vi "Caliper Setting UI.vi"(7 "Coor?":bool, 8 "error in (no error)":errorcluster, 9 "CaliperEntryIn Overlay In":T2[](array[typedef]) {"CaliperType" items=["Distance", "Mid Point", "Perpendicular Projection", "Lines Intersection", "Angle from Horizontal", "Angle from Vertical", "Angle Defined by 3 Points", "Angle Defined by 4 Points", "Bissecting Line", "Mid Line", "Center of Mass", "Area", "Line Fit", "Circle Fit", "Ellipse Fit"]}, 10 "CaliperEntryIn":T2[](array[typedef]) {"CaliperType" items=["Distance", "Mid Point", "Perpendicular Projection", "Lines Intersection", "Angle from Horizontal", "Angle from Vertical", "Angle Defined by 3 Points", "Angle Defined by 4 Points", "Bissecting Line", "Mid Line", "Center of Mass", "Area", "Line Fit", "Circle Fit", "Ellipse Fit"]}, 11 "Vision_Image":T7(plugin-control)) -> (0 "error out":errorcluster, 1 "CaliperEntryOut Overlay":T2[](array[typedef]) {"CaliperType" items=["Distance", "Mid Point", "Perpendicular Projection", "Lines Intersection", "Angle from Horizontal", "Angle from Vertical", "Angle Defined by 3 Points", "Angle Defined by 4 Points", "Bissecting Line", "Mid Line", "Center of Mass", "Area", "Line Fit", "Circle Fit", "Ellipse Fit"]}, 2 "CaliperEntryOut":T2[](array[typedef]) {"CaliperType" items=["Distance", "Mid Point", "Perpendicular Projection", "Lines Intersection", "Angle from Horizontal", "Angle from Vertical", "Angle Defined by 3 Points", "Angle Defined by 4 Points", "Bissecting Line", "Mid Line", "Center of Mass", "Area", "Line Fit", "Circle Fit", "Ellipse Fit"]}, 3 "Cancel?":bool)   [LabVIEW 2019]
uses:
  Controls/CaliperType with Picture.ctl
  Controls/SelectionListEntry.ctl
  Controls/SelectionListEntryPointType.ctl
  Controls/CaliperDataEntry.ctl
  Controls/CaliperType.ctl
  Controls/CaliperResult.ctl
  Controls/Caliper_UI_Action.ctl
  Controls/AnalysisResultPointsAction.ctl
  Analysis/Controls/Analysis_Result_To_Caliper.ctl
  <vilib>/vision/NI_Vision_Development_Module.lvlib
panel:
  out "Result Overlay":T1
  out "CaliperEntryList Overlay":T2[](array[typedef]) {"CaliperType" items=["Distance", "Mid Point", "Perpendicular Projection", "Lines Intersection", "Angle from Horizontal", "Angle from Vertical", "Angle Defined by 3 Points", "Angle Defined by 4 Points", "Bissecting Line", "Mid Line", "Center of Mass", "Area", "Line Fit", "Circle Fit", "Ellipse Fit"]}
  in  "Run All":bool
  in  "ReplaceCaliper":bool
  out "Result":string
  in  "DeleteCaliper":bool
  in  "CaliperList":i32(listbox)=-1
  in  "AddCaliper":bool
  out "Result":T1
  out "CaliperEntryList":T2[](array[typedef]) {"CaliperType" items=["Distance", "Mid Point", "Perpendicular Projection", "Lines Intersection", "Angle from Horizontal", "Angle from Vertical", "Angle Defined by 3 Points", "Angle Defined by 4 Points", "Bissecting Line", "Mid Line", "Center of Mass", "Area", "Line Fit", "Circle Fit", "Ellipse Fit"]}
  out "AnalysisResultNum":i32
  out "SelectionList":T4[](array[typedef])
  out "Row":i32
  out "Analysis Results":i32[](listbox)
  in  "CaliperType_w_Pic":T6 items=["Distance", "Mid Point", "Perpendicular Projection", "Lines Intersection", "Angle from Horizontal", "Angle from Vertical", "Angle Defined by 3 Points", "Angle Defined by 4 Points", "Bissecting Line", "Mid Line", "Area", "Line Fit", "Circle Fit"]
  in  "Cancel":bool
  in  "Done":bool
  in  "Run Algorithm":bool
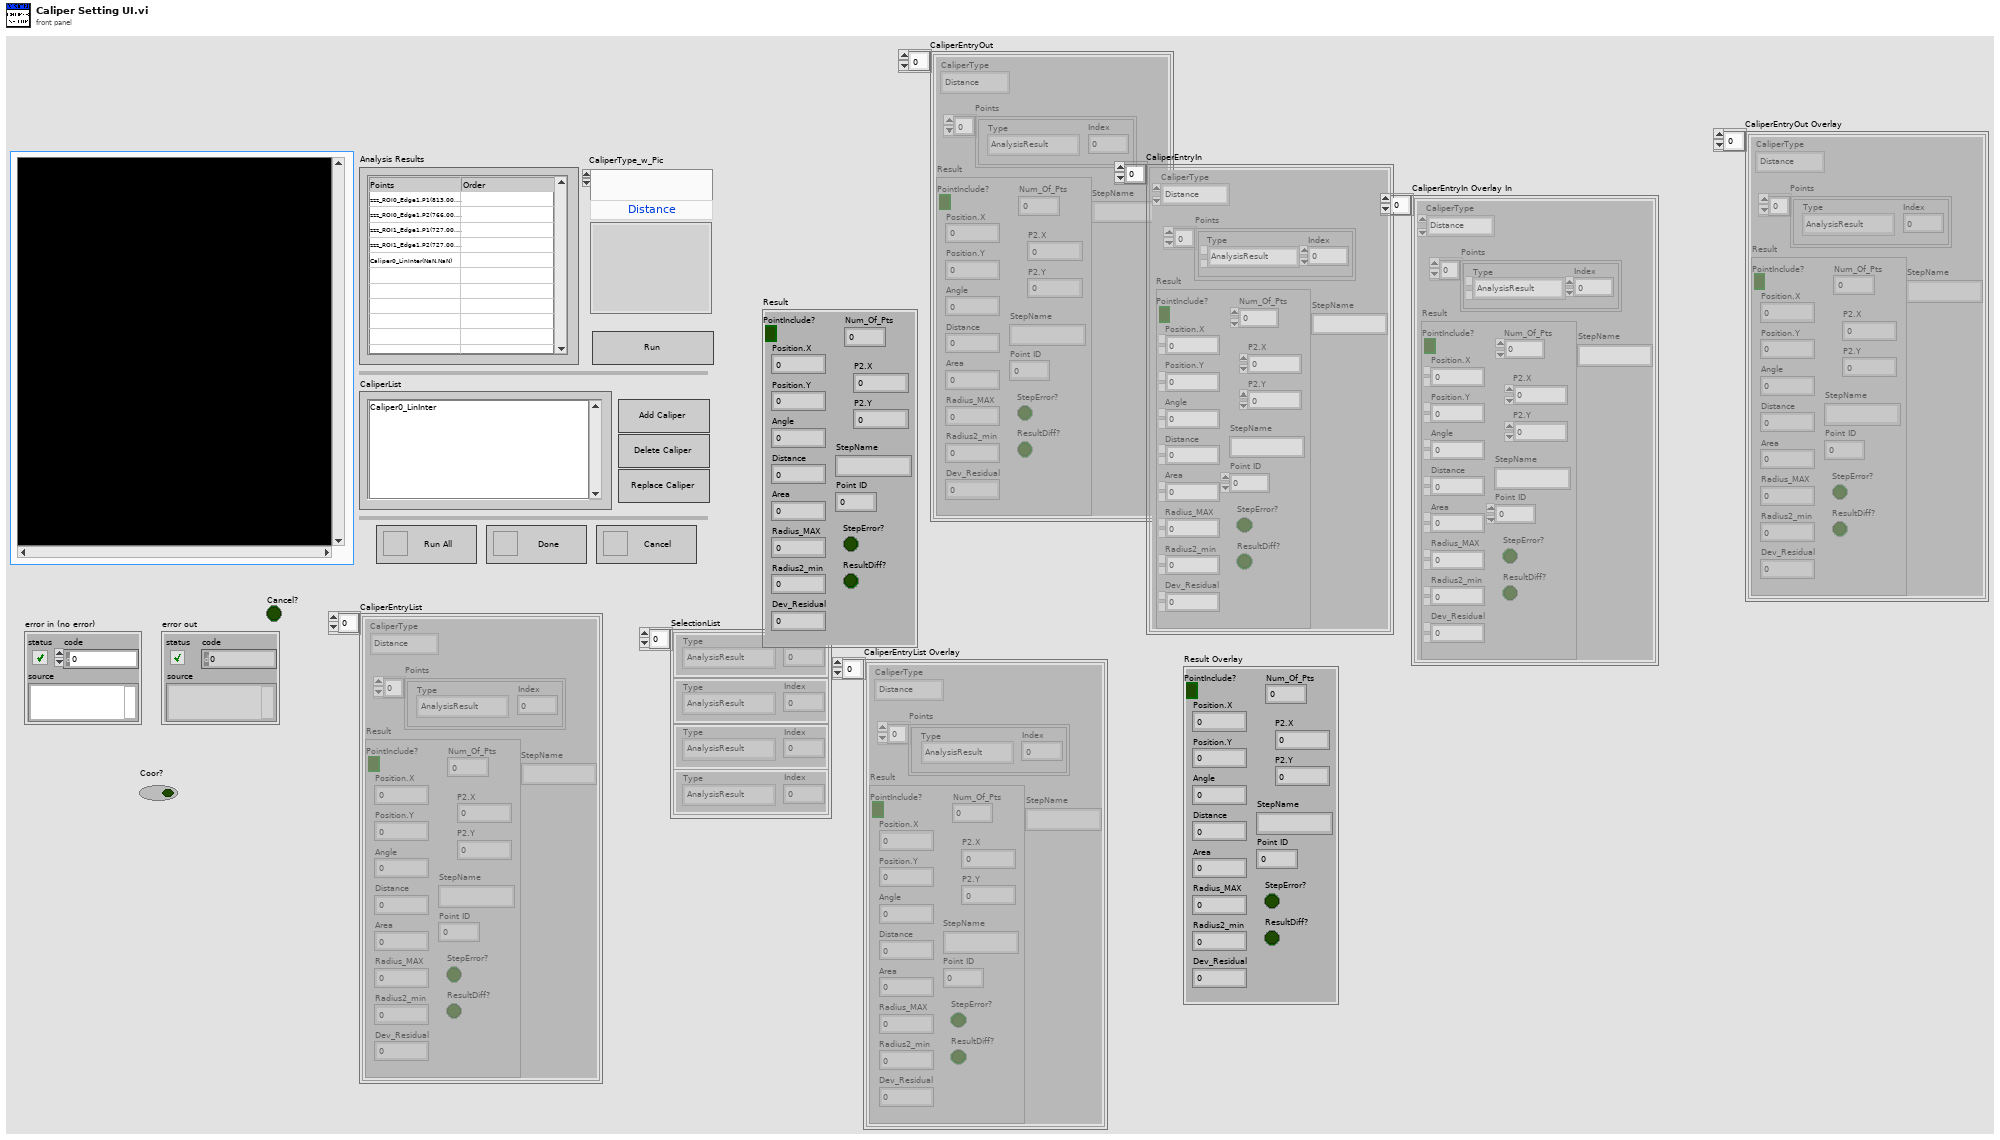
[diagram p1: front panel]
types:
  T1 = typedef "CaliperResult.ctl" = cluster{"PointInclude?":bool, "Num_Of_Pts":u8, "Position.X":dbl, "Position.Y":dbl, "Angle":dbl, "Distance":dbl, "Area":dbl, "Radius_MAX":dbl, "Radius2_min":dbl, "Dev_Residual":dbl, "P2.X":dbl, "P2.Y":dbl, "StepName":string, "Point ID":u8, "StepError?":bool, "ResultDiff?":bool}
  T2 = typedef "CaliperDataEntry.ctl" = cluster{"CaliperType":T3, "Points":T4[], "Result":T1, "StepName":string}
  T3 = typedef "CaliperType.ctl" = u32
  T4 = typedef "SelectionListEntry.ctl" = cluster{"Type":T5, "Index":i32}
  T5 = typedef "SelectionListEntryPointType.ctl" = enum16{"AnalysisResult", "CaliperResult"}
  T6 = typedef "CaliperType with Picture.ctl" = u32
  T7 = typedef "IMAQ Image.ctl" = refnum<image>
  T8 = typedef "Caliper_UI_Action.ctl" = enum16{"Init", "Done", "Cancel", "Run", "InitAnalysisResultTable", "UpdateSymbol", "UpdateOrderInTable", "UpdateAnalysisTable", "UpdateCaliperResultToTable", "AddCaliperEntry", "SetCaliperStepName", "UpdateCaliperList", "RemoveCaliperEntry", "ResetSelectionList", "ReplaceCaliperEntry", "RunAll", "Updata Overlay", "Clean Overlay"}
  T9 = typedef "Analysis_Result_To_Caliper.ctl" = cluster{"PointName":string, "Position_X":dbl, "Position_Y":dbl}
  T10 = typedef "AnalysisResultPointsAction.ctl" = enum16{"Init", "Add", "Delete", "ReplaceAll", "ReadAll", "Close"}
  T11 = typedef "CaliperDataEntry_SinglePoint.ctl" = cluster{"CaliperType":T3, "Points":T4[], "Result":T12, "StepName":string}
  T12 = typedef "CaliperResult_SinglePoint.ctl" = cluster{"PointInclude?":bool, "Position.X":dbl, "Position.Y":dbl, "Angle":dbl, "Distance":dbl, "Area":dbl, "Radius_MAX":dbl, "Radius2_min":dbl, "Dev_Residual":dbl, "StepName":string, "Point ID":u8, "StepError?":bool, "ResultDiff?":bool}
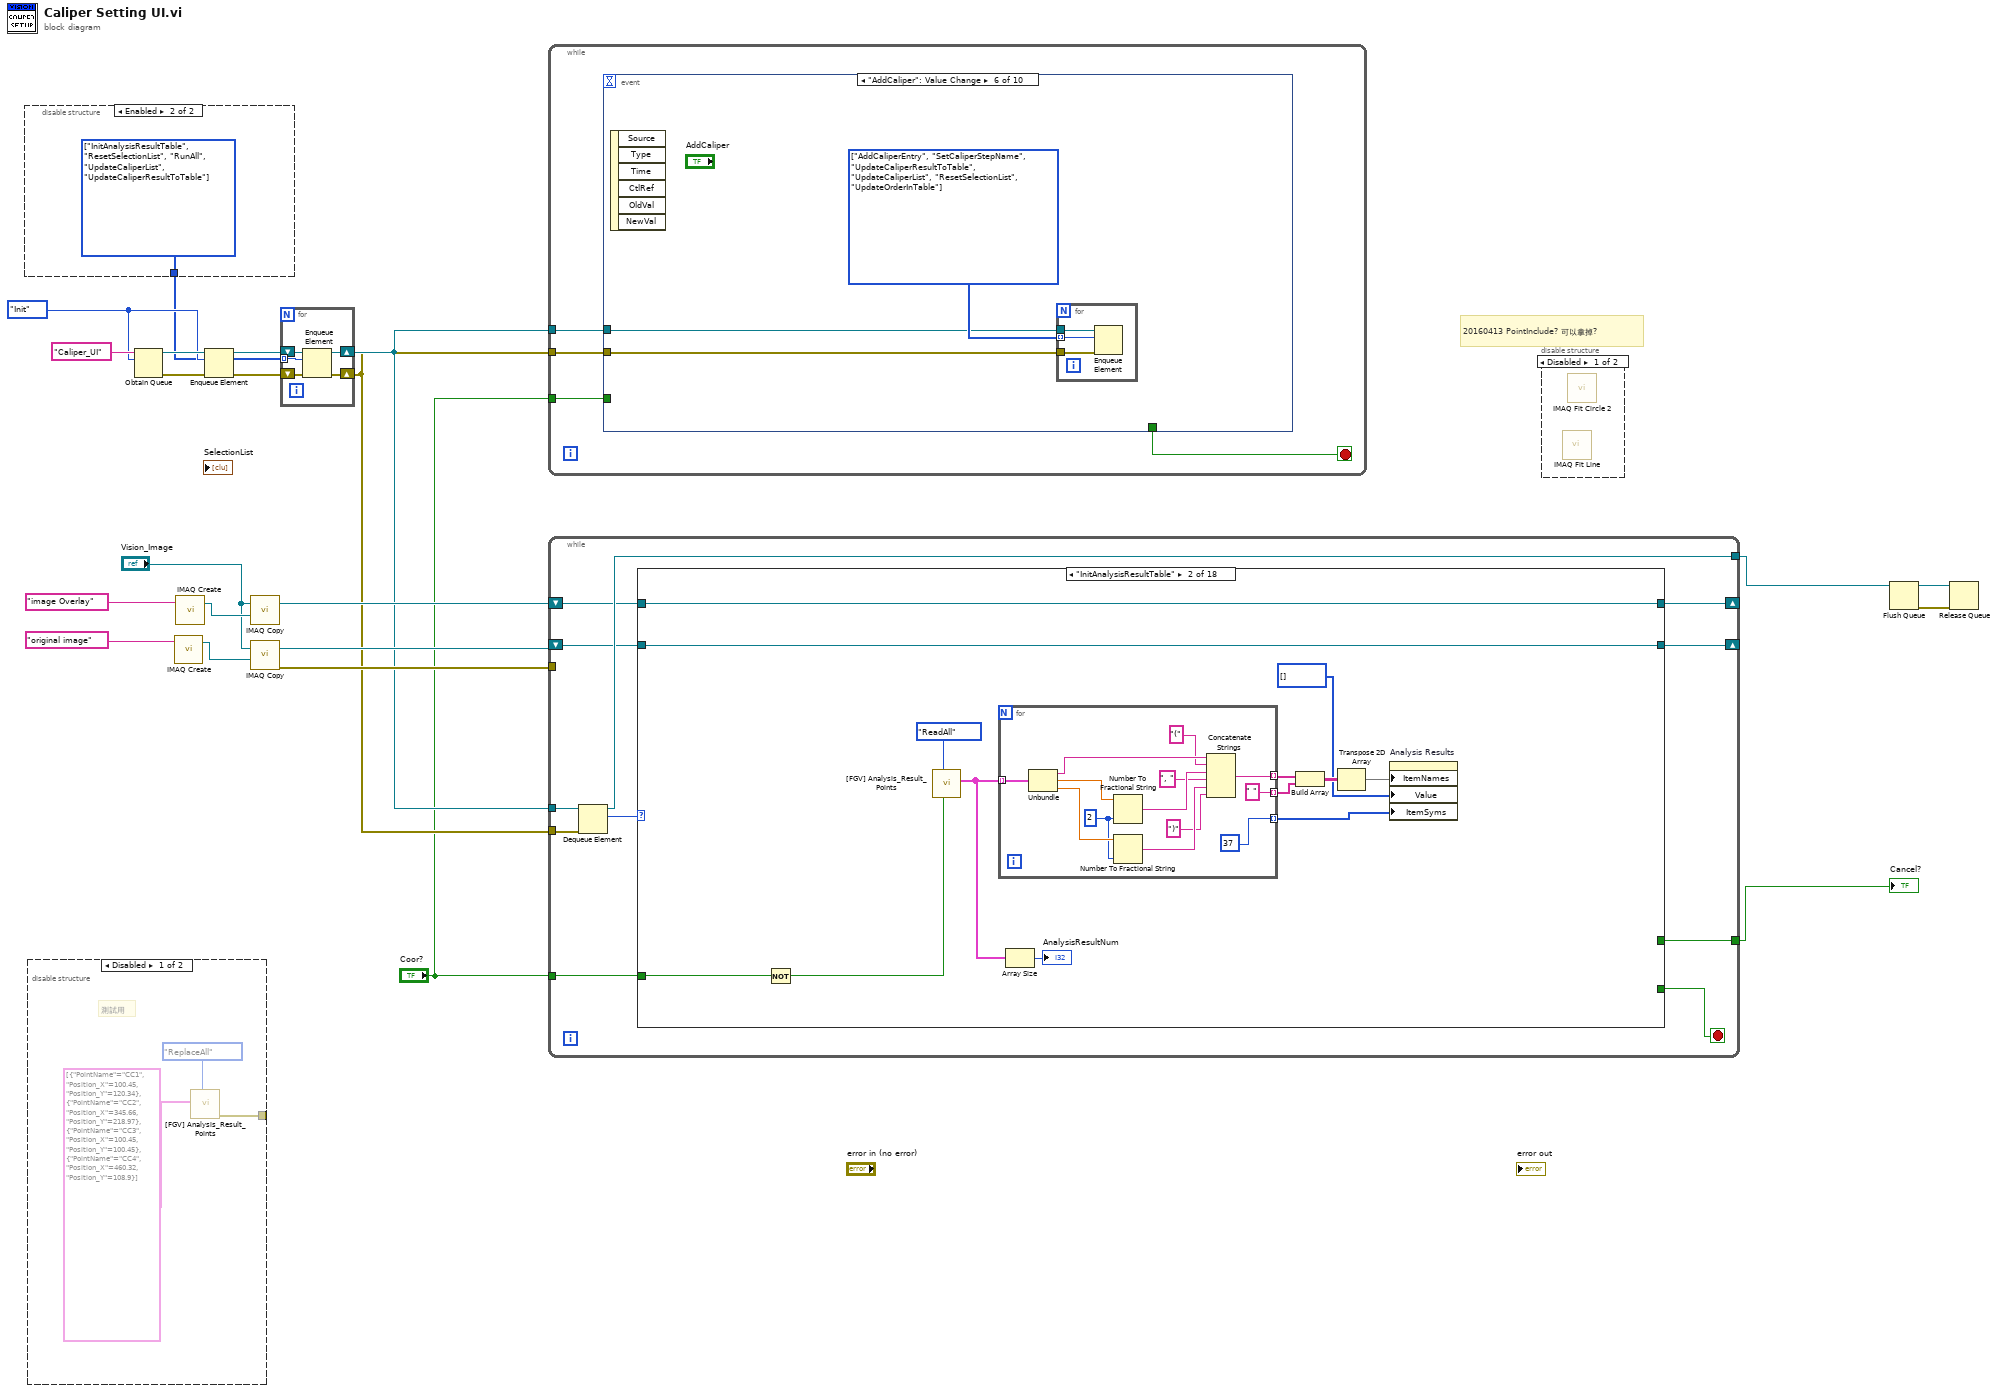
[diagram p0: block diagram]
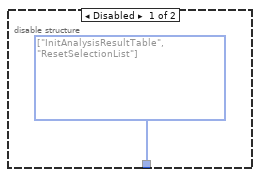
[diagram p3: hidden frame]
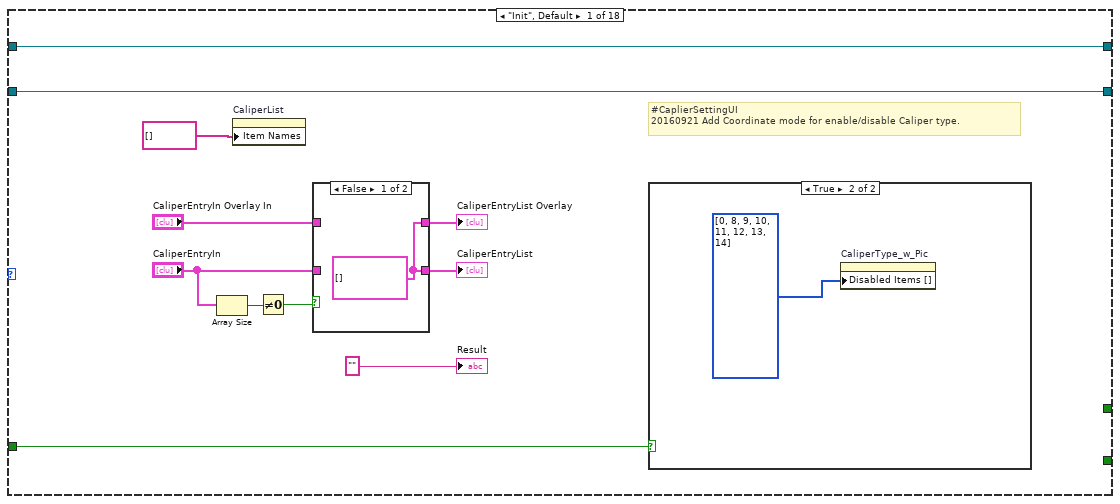
[diagram p5: hidden frame]
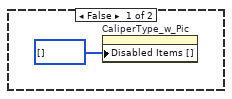
[diagram p6: hidden frame]
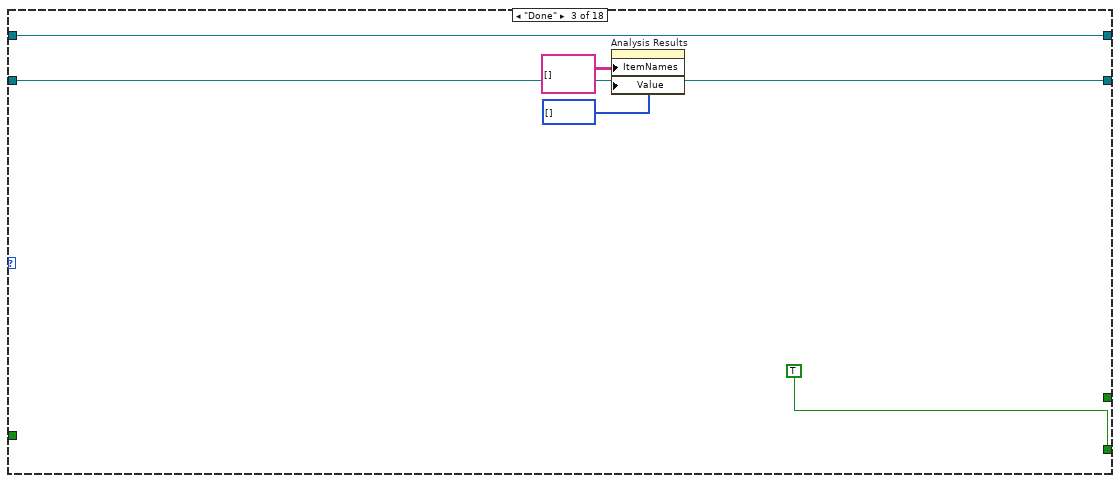
[diagram p8: hidden frame]
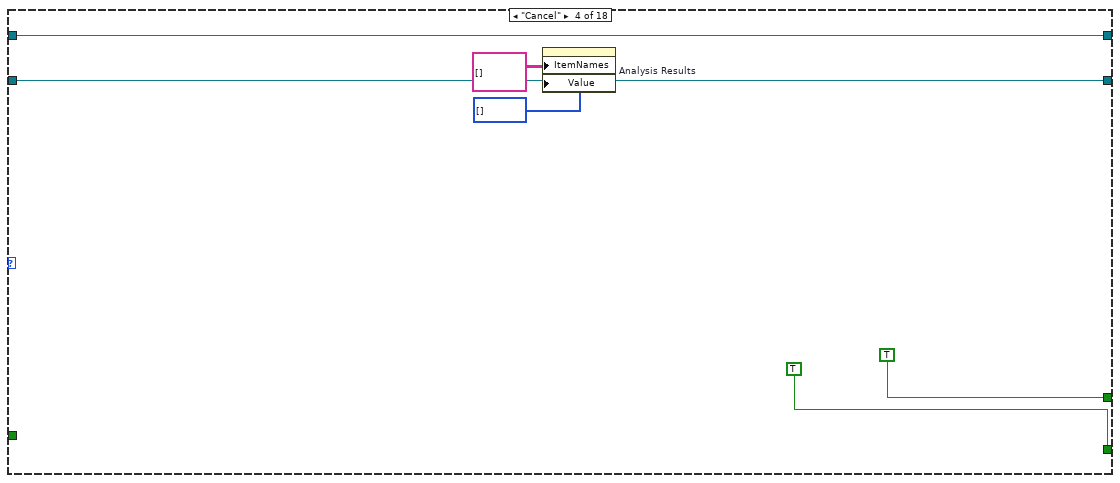
[diagram p9: hidden frame]
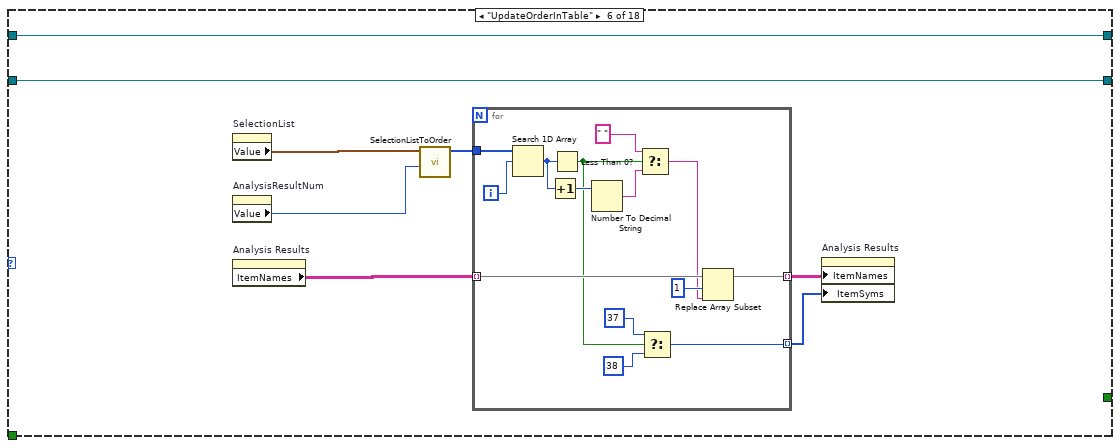
[diagram p11: hidden frame]
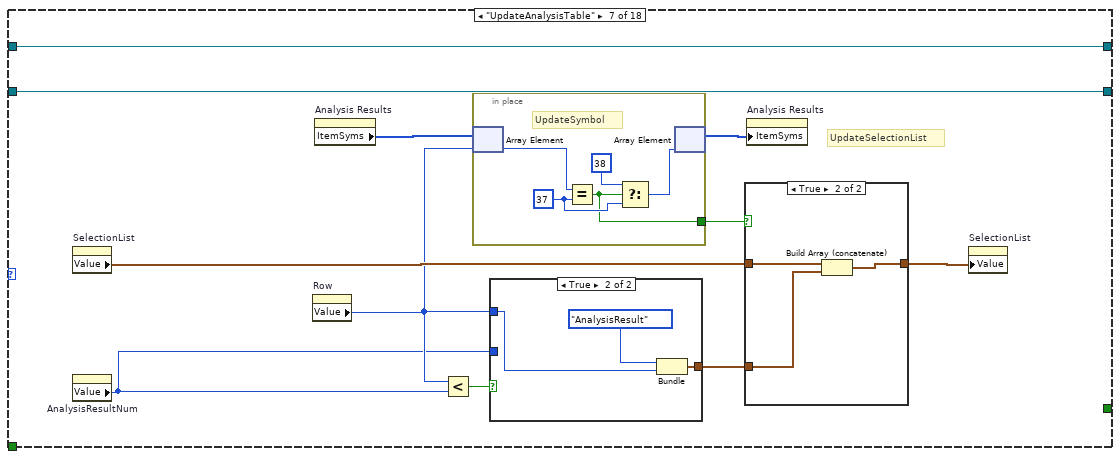
[diagram p12: hidden frame]
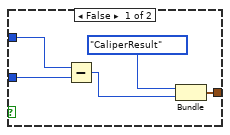
[diagram p13: hidden frame]
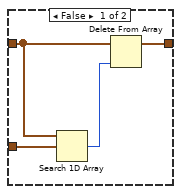
[diagram p14: hidden frame]
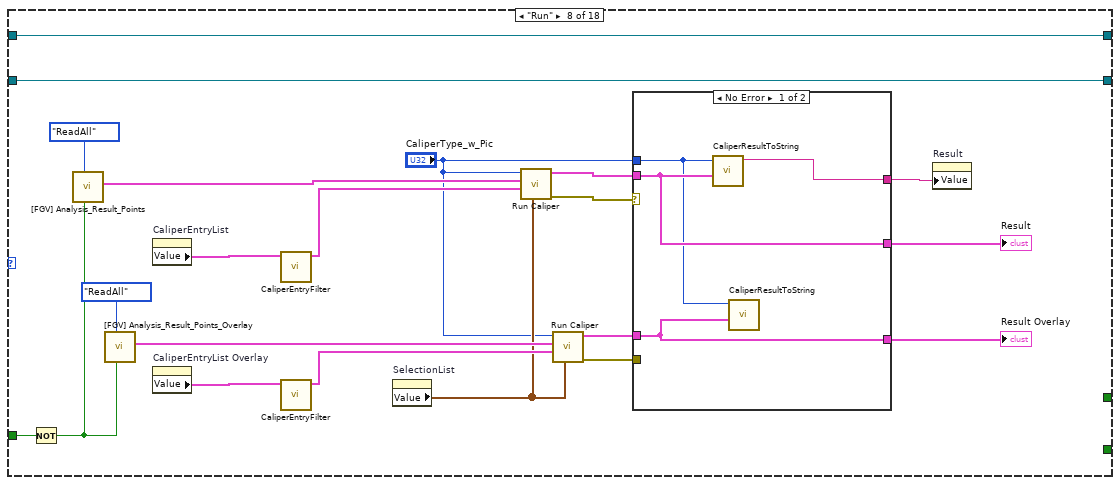
[diagram p15: hidden frame]
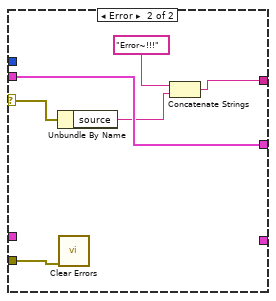
[diagram p16: hidden frame]
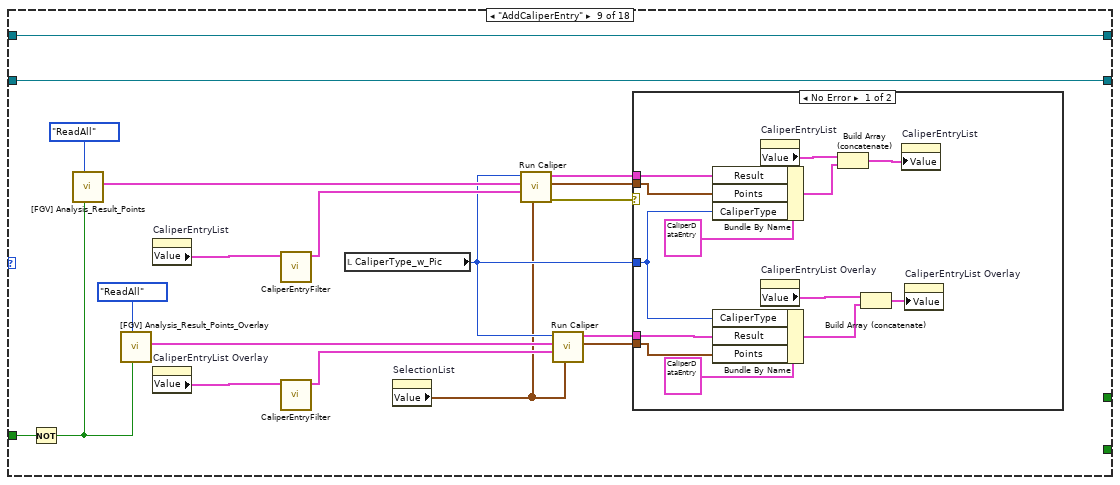
[diagram p17: hidden frame]
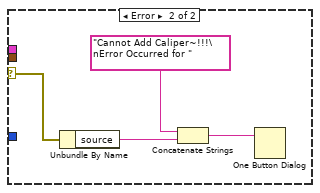
[diagram p18: hidden frame]
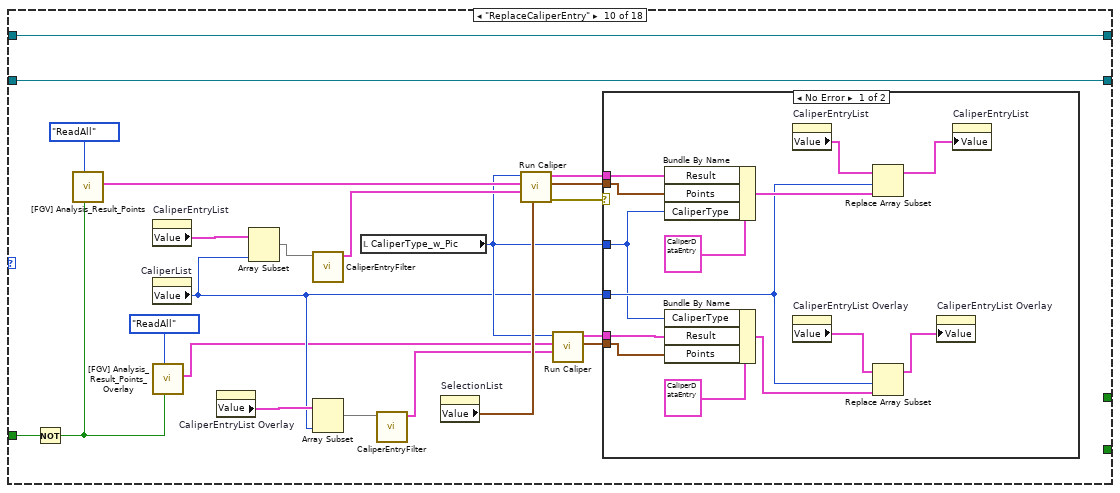
[diagram p19: hidden frame]
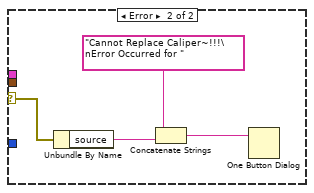
[diagram p20: hidden frame]
diagram:
  w20 = Caliper_UI_Action."Init" ("CaliperAction")
  # "20160413 PointInclude? 可以拿掉?"
  n1 = disable-structure shown="Enabled" {
    disable-tunnel: [w23 w24] -> w12
    frame Disabled {
      w23 = T8[] [enum."InitAnalysisResultTable", enum."ResetSelectionList"] items=["Init", "Done", "Cancel", "Run", "InitAnalysisResultTable", "UpdateSymbol", "UpdateOrderInTable", "UpdateAnalysisTable", "UpdateCaliperResultToTable", "AddCaliperEntry", "SetCaliperStepName", "UpdateCaliperList", "RemoveCaliperEntry", "ResetSelectionList", "ReplaceCaliperEntry", "RunAll", "Updata Overlay", "Clean Overlay"]
    }
    frame Enabled {
      w24 = T8[] [enum."InitAnalysisResultTable", enum."ResetSelectionList", enum."RunAll", enum."UpdateCaliperList", enum."UpdateCaliperResultToTable"] items=["Init", "Done", "Cancel", "Run", "InitAnalysisResultTable", "UpdateSymbol", "UpdateOrderInTable", "UpdateAnalysisTable", "UpdateCaliperResultToTable", "AddCaliperEntry", "SetCaliperStepName", "UpdateCaliperList", "RemoveCaliperEntry", "ResetSelectionList", "ReplaceCaliperEntry", "RunAll", "Updata Overlay", "Clean Overlay"]
    }
  }
  n2 = disable-structure shown="Disabled" {
    disable-tunnel: [w26 _] -> _
    frame Disabled {
      # "測試用"
      n3 = call "[FGV] Analysis_Result_Points.vi"("Action"=AnalysisResultPointsAction."ReplaceAll", "Analysis_Point_Result"=T9[] [{"PointName"="CC1", "Position_X"=100.45, "Position_Y"=120.34}, {"PointName"="CC2", "Position_X"=345.66, "Position_Y"=218.97}, {"PointName"="CC3", "Position_X"=100.45, "Position_Y"=100.45}, {"PointName"="CC4", "Position_X"=460.32, "Position_Y"=108.9}]) -> ("error out"=w26:errorcluster)  [unwired: 8 in, 1 out]
    }
    frame Enabled {
    }
  }
  n4 = Obtain Queue(name (unnamed)="Caliper_UI", element data type=w20) -> (queue out=w21:refnum<queue>, error out=w15:errorcluster)  [unwired: 3 in, 1 out]
  n5 = call "IMAQ Create"("Image Name"="original image") -> ("New Image"=w8:T7)  [unwired: 4 in, 1 out]
  n6 = call "IMAQ Create"("Image Name"="image Overlay") -> ("New Image"=w11:T7)  [unwired: 4 in, 1 out]
  n7 = Enqueue Element(queue=w21, element=w20, error in (no error)=w15) -> (queue out=w14:refnum<queue>, error out=w13:errorcluster)  [unwired: 1 in, 1 out]
  n8 = call "IMAQ Copy"("Image Dst"=w11, "Image Src"="Vision_Image") -> ("Image Dst Out"=w5:T7)  [unwired: 4 in, 1 out]
  n9 = call "IMAQ Copy"("Image Dst"=w8, "Image Src"="Vision_Image") -> ("error out"=w6:errorcluster, "Image Dst Out"=w4:T7)  [unwired: 4 in]
  n10 = for {
    tunnel: w12 -> [w28] mode=indexing
    shift-right: [w31] -> w3
    shift-left: w14 -> [w32]
    shift-right: [w29] -> w2
    shift-left: w13 -> [w30]
    n11 = Enqueue Element(queue=w32, element=w28, error in (no error)=w30) -> (queue out=w31:refnum<queue>, error out=w29:errorcluster)  [unwired: 1 in, 1 out]
  }
  n12 = while {
    tunnel: w3 -> [w36]
    tunnel: w2 -> [w35]
    tunnel: "Coor?" -> [w33]
    stop <- w34 stop-if-true
    n13 = event shown="[5] \"AddCaliper\": Value Change" {
      selector: _ -> [_ _ _ _ _ _ _ _ _ _]
      dyn-events: _ -> [_ _ _ _ _ _ _ _ _ _]
      timeout: _ -> [_ _ _ _ _ _ _ _ _ _]
      tunnel: w36 -> [_ w45 w70 w76 w86 w91 w99 w117 w131 w141]
      tunnel: w35 -> [_ w44 w69 w75 w85 w90 w98 w116 _ w140]
      tunnel: [_ w46 TRUE _ _ _ _ _ _ _] -> w34
      tunnel: w33 -> [_ w39 _ _ _ _ _ _ _ _]
      event Timeout {
        n14 = event-data() -> ()  [unwired: 1 in, 2 out]
      }
      event "Done": Value Change {
        n15 = event-data() -> ()  [unwired: 1 in, 6 out]
        n16 = Not(x=w39) -> (.not. x?=w38:bool)
        n17 = call "[FGV] Analysis_Result_Points.vi"("CoordSystemRun"=w38, "Action"=AnalysisResultPointsAction."ReadAll") -> ("Analysis_Point_Result Out"=w49:T9[])  [unwired: 8 in, 1 out]
        n18 = property on="CaliperEntryList" class="Arr (strict)"() -> ("Value"=w50:T2[])  [unwired: 2 in, 2 out]
        n19 = call "[FGV] Analysis_Result_Points_Overlay.vi"("CoordSystemRun"=w38, "Action"=AnalysisResultPointsAction."ReadAll") -> ("Analysis_Point_Result Out"=w41:T9[])  [unwired: 8 in, 1 out]
        n20 = property on="CaliperEntryList Overlay" class="Arr (strict)"() -> ("Value"=w42:T2[])  [unwired: 2 in, 2 out]
        n21 = disable-structure shown="Disabled" {
          disable-tunnel: w50 -> [w53 w54]
          disable-tunnel: [w52 w54] -> w37
          frame Disabled {
            n22 = call "CaliperEntrySetToNone.vi"("CaliperEntryList"=w53) -> ("CaliperEntryOut"=w52:T2[])  [unwired: 9 in, 1 out]
          }
          frame Enabled {
          }
        }
        n23 = call "Check All Caliper Steps.vi"("Analysis_Point_Result"=w49, "CaliperEntryList"=w37) -> ("error out"=w48:errorcluster, "Index"=w47:i32)  [unwired: 7 in, 1 out]
        n24 = call "Check All Caliper Steps.vi"("Analysis_Point_Result"=w41, "CaliperEntryList"=w42) -> ("CaliperEntryOut"=w40:T2[])  [unwired: 7 in, 2 out]
        n25 = case shown="No Error" w48 {
          tunnel: [TRUE FALSE] -> w46
          tunnel: w37 -> [w59 _]
          tunnel: w47 -> [_ w64]
          tunnel: w45 -> [w57 _]
          tunnel: w44 -> [w56 _]
          tunnel: w40 -> [w55 _]
          frame No Error {
            n26 = Enqueue Element(queue=w57, element=Caliper_UI_Action."Done", error in (no error)=w56) -> ()  [unwired: 1 in, 3 out]
            "CaliperEntryOut" <- w59
            "CaliperEntryOut Overlay" <- w55
          }
          frame Error {
            n27 = Number To Decimal String(number=w64) -> (decimal integer string=w63:string)  [unwired: 1 in]
            n28 = Concatenate Strings("Error Occurred at Caliper", w63, ", Please Check Your Setting" ("string")) -> (w61:string)
            n29 = One Button Dialog(message=w61) -> ()  [unwired: 1 in, 1 out]
          }
        }
      }
      event "Cancel": Value Change {
        n30 = event-data() -> ()  [unwired: 1 in, 6 out]
        n31 = Enqueue Element(queue=w70, element=Caliper_UI_Action."Cancel", error in (no error)=w69) -> ()  [unwired: 1 in, 3 out]
      }
      event "Analysis Results": Double Click {
        n32 = event-data() -> ("CtlRef"=w77:refnum<vi>, "Row"=w73:i32)  [unwired: 1 in, 7 out]
        "Row" <- w73
        n33 = property class="MCListbox (strict)"(reference=w77) -> ("ItemSyms"=w74:i32[])  [unwired: 1 in, 2 out]
        n34 = Array Size(array=w74) -> (size(s)=w72:i32)
        n35 = Less?(x=w73, y=w72) -> (x < y?=w71:bool)
        n36 = case shown="True" w71 {
          tunnel: w76 -> [_ w80]
          tunnel: w75 -> [_ w79]
          frame False {
          }
          frame True {
            w78 = T8[] [enum."UpdateSymbol", enum."UpdateAnalysisTable", enum."UpdateOrderInTable"] items=["Init", "Done", "Cancel", "Run", "InitAnalysisResultTable", "UpdateSymbol", "UpdateOrderInTable", "UpdateAnalysisTable", "UpdateCaliperResultToTable", "AddCaliperEntry", "SetCaliperStepName", "UpdateCaliperList", "RemoveCaliperEntry", "ResetSelectionList", "ReplaceCaliperEntry", "RunAll", "Updata Overlay", "Clean Overlay"]
            n37 = for {
              tunnel: w80 -> [w83]
              tunnel: w79 -> [w82]
              tunnel: w78 -> [w81] mode=indexing
              n38 = Enqueue Element(queue=w83, element=w81, error in (no error)=w82) -> ()  [unwired: 1 in, 3 out]
            }
          }
        }
      }
      event "Run Algorithm": Value Change {
        w84 = T8[] [enum."Run", enum."Clean Overlay", enum."Updata Overlay"] items=["Init", "Done", "Cancel", "Run", "InitAnalysisResultTable", "UpdateSymbol", "UpdateOrderInTable", "UpdateAnalysisTable", "UpdateCaliperResultToTable", "AddCaliperEntry", "SetCaliperStepName", "UpdateCaliperList", "RemoveCaliperEntry", "ResetSelectionList", "ReplaceCaliperEntry", "RunAll", "Updata Overlay", "Clean Overlay"]
        n39 = event-data() -> ()  [unwired: 1 in, 6 out]
        n40 = for {
          tunnel: w86 -> [w89]
          tunnel: w85 -> [w88]
          tunnel: w84 -> [w87] mode=indexing
          n41 = Enqueue Element(queue=w89, element=w87, error in (no error)=w88) -> ()  [unwired: 1 in, 3 out]
        }
      }
      event "AddCaliper": Value Change {
        w92 = T8[] [enum."AddCaliperEntry", enum."SetCaliperStepName", enum."UpdateCaliperResultToTable", enum."UpdateCaliperList", enum."ResetSelectionList", enum."UpdateOrderInTable"] items=["Init", "Done", "Cancel", "Run", "InitAnalysisResultTable", "UpdateSymbol", "UpdateOrderInTable", "UpdateAnalysisTable", "UpdateCaliperResultToTable", "AddCaliperEntry", "SetCaliperStepName", "UpdateCaliperList", "RemoveCaliperEntry", "ResetSelectionList", "ReplaceCaliperEntry", "RunAll", "Updata Overlay", "Clean Overlay"]
        n42 = event-data() -> ()  [unwired: 1 in, 6 out]
        n43 = for {
          tunnel: w90 -> [w95]
          tunnel: w91 -> [w94]
          tunnel: w92 -> [w93] mode=indexing
          n44 = Enqueue Element(queue=w94, element=w93, error in (no error)=w95) -> ()  [unwired: 1 in, 3 out]
        }
      }
      event "DeleteCaliper": Value Change {
        n45 = event-data() -> ()  [unwired: 1 in, 6 out]
        n46 = property on="CaliperList" class="LstBox (strict)"() -> ("Value"=w97:i32)  [unwired: 2 in, 2 out]
        n47 = Greater Or Equal To 0?(x=w97) -> (x >= 0?=w96:bool)
        n48 = case shown="False" w96 {
          tunnel: w99 -> [_ w102]
          tunnel: w98 -> [_ w101]
          frame False {
          }
          frame True {
            # "20160413\nadd step\n\"Run All\"\nfor update\nCaliper Result"
            n49 = disable-structure shown="Enabled" {
              disable-tunnel: [w103 w104] -> w100
              frame Disabled {
                w103 = T8[] [enum."RemoveCaliperEntry", enum."SetCaliperStepName", enum."UpdateCaliperResultToTable", enum."UpdateCaliperList", enum."ResetSelectionList", enum."UpdateOrderInTable"] items=["Init", "Done", "Cancel", "Run", "InitAnalysisResultTable", "UpdateSymbol", "UpdateOrderInTable", "UpdateAnalysisTable", "UpdateCaliperResultToTable", "AddCaliperEntry", "SetCaliperStepName", "UpdateCaliperList", "RemoveCaliperEntry", "ResetSelectionList", "ReplaceCaliperEntry", "RunAll", "Updata Overlay", "Clean Overlay"]
              }
              frame Enabled {
                w104 = T8[] [enum."RemoveCaliperEntry", enum."SetCaliperStepName", enum."RunAll", enum."UpdateCaliperResultToTable", enum."UpdateCaliperList", enum."ResetSelectionList", enum."UpdateOrderInTable"] items=["Init", "Done", "Cancel", "Run", "InitAnalysisResultTable", "UpdateSymbol", "UpdateOrderInTable", "UpdateAnalysisTable", "UpdateCaliperResultToTable", "AddCaliperEntry", "SetCaliperStepName", "UpdateCaliperList", "RemoveCaliperEntry", "ResetSelectionList", "ReplaceCaliperEntry", "RunAll", "Updata Overlay", "Clean Overlay"]
              }
            }
            n50 = for {
              tunnel: w101 -> [w107]
              tunnel: w102 -> [w106]
              tunnel: w100 -> [w105] mode=indexing
              n51 = Enqueue Element(queue=w106, element=w105, error in (no error)=w107) -> ()  [unwired: 1 in, 3 out]
            }
          }
        }
      }
      event "ReplaceCaliper": Value Change {
        n52 = event-data() -> ()  [unwired: 1 in, 6 out]
        n53 = local read "CaliperType_w_Pic"() -> (w109:T6)
        n54 = property on="CaliperList" class="LstBox (strict)"() -> ("Value"=w112:i32)  [unwired: 2 in, 2 out]
        n55 = property on="CaliperEntryList" class="Arr (strict)"() -> ("Value"=w113:T2[])  [unwired: 2 in, 2 out]
        n56 = Index Array(array=w113, index=w112) -> (element=w111:T2)
        n57 = Greater Or Equal To 0?(x=w112) -> (x >= 0?=w114:bool)
        n58 = Unbundle By Name(w111) -> ("CaliperType"=w110:T3)
        n59 = Equal?(x=w110, y=w109) -> (x = y?=w108:bool)
        n60 = And(x=w114, y=w108) -> (x .and. y?=w115:bool)
        n61 = case shown="True" w115 {
          tunnel: w117 -> [_ w122]
          tunnel: w116 -> [_ w121]
          tunnel: w108 -> [w118 _]
          frame False {
            n62 = case shown="False" w118 {
              frame False {
                n63 = One Button Dialog(message="Caliper Type Must Be Equal To Change Caliper Entry") -> ()  [unwired: 1 in, 1 out]
              }
              frame True {
              }
            }
          }
          frame True {
            n64 = disable-structure shown="Enabled" {
              disable-tunnel: [w123 w124] -> w120
              frame Enabled {
                w123 = T8[] [enum."ReplaceCaliperEntry", enum."SetCaliperStepName", enum."UpdateCaliperResultToTable", enum."UpdateCaliperList", enum."UpdateOrderInTable"] items=["Init", "Done", "Cancel", "Run", "InitAnalysisResultTable", "UpdateSymbol", "UpdateOrderInTable", "UpdateAnalysisTable", "UpdateCaliperResultToTable", "AddCaliperEntry", "SetCaliperStepName", "UpdateCaliperList", "RemoveCaliperEntry", "ResetSelectionList", "ReplaceCaliperEntry", "RunAll", "Updata Overlay", "Clean Overlay"]
              }
              frame Disabled {
                w124 = T8[] [enum."ReplaceCaliperEntry"] items=["Init", "Done", "Cancel", "Run", "InitAnalysisResultTable", "UpdateSymbol", "UpdateOrderInTable", "UpdateAnalysisTable", "UpdateCaliperResultToTable", "AddCaliperEntry", "SetCaliperStepName", "UpdateCaliperList", "RemoveCaliperEntry", "ResetSelectionList", "ReplaceCaliperEntry", "RunAll", "Updata Overlay", "Clean Overlay"]
              }
            }
            n65 = for {
              tunnel: w121 -> [w127]
              tunnel: w122 -> [w126]
              tunnel: w120 -> [w125] mode=indexing
              n66 = Enqueue Element(queue=w126, element=w125, error in (no error)=w127) -> ()  [unwired: 1 in, 3 out]
            }
          }
        }
      }
      event "CaliperList": Value Change {
        w128 = T8[] [enum."UpdateOrderInTable", enum."Clean Overlay"] items=["Init", "Done", "Cancel", "Run", "InitAnalysisResultTable", "UpdateSymbol", "UpdateOrderInTable", "UpdateAnalysisTable", "UpdateCaliperResultToTable", "AddCaliperEntry", "SetCaliperStepName", "UpdateCaliperList", "RemoveCaliperEntry", "ResetSelectionList", "ReplaceCaliperEntry", "RunAll", "Updata Overlay", "Clean Overlay"]
        n67 = event-data() -> ("NewVal"=w134:i32)  [unwired: 1 in, 1 out]
        n68 = property on="CaliperEntryList" class="Arr (strict)"() -> ("Value"=w135:T2[])  [unwired: 2 in, 2 out]
        n69 = Index Array(array=w135, index=w134) -> (element=w133:T2)
        n70 = Unbundle By Name(w133) -> ("CaliperType"=w129:T3, "Points"=w132:T4[])
        n71 = property on="CaliperType_w_Pic" class="Ring (strict)"("Value"=w129) -> ()  [unwired: 2 in, 2 out]
        n72 = property on="SelectionList" class="Arr (strict)"("Value"=w132) -> (error out=w130:errorcluster)  [unwired: 2 in, 1 out]
        n73 = for {
          tunnel: w131 -> [w138]
          tunnel: w130 -> [w137]
          tunnel: w128 -> [w136] mode=indexing
          n74 = Enqueue Element(queue=w138, element=w136, error in (no error)=w137) -> ()  [unwired: 1 in, 3 out]
        }
      }
      event "Run All": Value Change {
        n75 = event-data() -> ()  [unwired: 1 in, 6 out]
        n76 = Enqueue Element(queue=w141, element=Caliper_UI_Action."RunAll", error in (no error)=w140) -> ()  [unwired: 1 in, 3 out]
      }
    }
  }
  n77 = while {
    tunnel: w3 -> [w152]
    tunnel: w2 -> [w151]
    tunnel: [w149] -> w19
    tunnel: [w148] -> w16
    tunnel: w6 -> [_]
    shift-right: [w144] -> _
    shift-left: w5 -> [w147]
    shift-right: [w145] -> _
    shift-left: w4 -> [w146]
    tunnel: "Coor?" -> [w142]
    stop <- w143 stop-if-true
    n78 = Dequeue Element(queue=w152, error in (no error)=w151) -> (queue out=w149:refnum<queue>, element=w150:T8)  [unwired: 1 in, 2 out]
    n79 = case shown="\"InitAnalysisResultTable\"" w150 {
      tunnel: [_ _ TRUE TRUE _ _ _ _ _ _ _ _ _ _ _ _ _ _] -> w143
      tunnel: [_ _ _ TRUE _ _ _ _ _ _ _ _ _ _ _ _ _ _] -> w148
      tunnel: w147 -> [w156 w172 w196 w201 w207 w209 w231 w273 w303 w340 w370 w399 w446 w459 w469 w482 w496 w512]
      tunnel: [w157 w171 w195 w200 w206 w208 w230 w272 w302 w339 w369 w398 w445 w458 w468 w481 w495 w513] -> w145
      tunnel: w146 -> [w157 w171 w195 w200 w206 w208 w230 w272 w302 w339 w369 w398 w445 w458 w468 w481 w495 w513]
      tunnel: [w156 w172 w196 w201 w207 w209 w231 w273 w303 w340 w370 w399 w446 w459 w469 w482 w494 w511] -> w144
      tunnel: w142 -> [w153 w170 _ _ _ _ _ w262 w293 w329 w368 _ _ _ _ w476 w492 _]
      frame "Init", Default {
        # "#CaplierSettingUI\n20160921 Add Coordinate mode for enable/disable Caliper type."
        n80 = Array Size(array="CaliperEntryIn") -> (size(s)=w161:i32)
        n81 = property on="CaliperList" class="LstBox (strict)"("Item Names"=string[] []) -> ()  [unwired: 2 in, 2 out]
        n82 = Not Equal To 0?(x=w161) -> (x != 0?=w160:bool)
        n83 = case shown="False" w160 {
          tunnel: "CaliperEntryIn" -> [_ w168]
          tunnel: [w166 w168] -> w158
          tunnel: [w166 w167] -> w155
          tunnel: "CaliperEntryIn Overlay In" -> [_ w167]
          frame False {
            w166 = T2[] [] ("CaliperEntryList")
          }
          frame True {
          }
        }
        "CaliperEntryList" <- w158
        "CaliperEntryList Overlay" <- w155
        n84 = case shown="True" w153 {
          frame False {
            n85 = property on="CaliperType_w_Pic" class="Ring (strict)"("Disabled Items []"=i32[] []) -> ()  [unwired: 2 in, 2 out]
          }
          frame True {
            n86 = property on="CaliperType_w_Pic" class="Ring (strict)"("Disabled Items []"=i32[] [0, 8, 9, 10, 11, 12, 13, 14]) -> ()  [unwired: 2 in, 2 out]
          }
        }
        "Result" <- "" ("Result")
      }
      frame "InitAnalysisResultTable" {
        n87 = Not(x=w170) -> (.not. x?=w169:bool)
        n88 = call "[FGV] Analysis_Result_Points.vi"("CoordSystemRun"=w169, "Action"=AnalysisResultPointsAction."ReadAll") -> ("Analysis_Point_Result Out"=w174:T9[])  [unwired: 8 in, 1 out]
        n89 = for {
          tunnel: w174 -> [w194] mode=indexing
          tunnel: [w184] -> w180 mode=indexing
          tunnel: [37] -> w179 mode=indexing
          tunnel: [" " ("string")] -> w175 mode=indexing
          w188 = i16 2 ("precision (6)")
          n90 = Unbundle(w194) -> ("PointName"=w191:string, "Position_X"=w193:dbl, "Position_Y"=w192:dbl)
          n91 = Number To Fractional String(number=w193, precision (6)=w188) -> (F-format string=w189:string)  [unwired: 2 in]
          n92 = Number To Fractional String(number=w192, precision (6)=w188) -> (F-format string=w186:string)  [unwired: 2 in]
          n93 = Concatenate Strings(w191, "(" ("string"), w189, ", " ("string"), w186, ")" ("string")) -> (w184:string)
        }
        n94 = Array Size(array=w174) -> (size(s)=→"AnalysisResultNum":i32)
        n95 = Build Array(w180, w175) -> (w178:string[][])
        n96 = Transpose 2D Array(2D array=w178) -> (transposed array=w176:string[][])
        n97 = property on="Analysis Results" class="MCListbox (strict)"("ItemNames"=w176, "Value"=i32[] [] ("Analysis Results"), "ItemSyms"=w179) -> ()  [unwired: 2 in, 2 out]
      }
      frame "Done" {
        n98 = property on="Analysis Results" class="MCListbox (strict)"("ItemNames"=string[][] [] ("Item Names"), "Value"=i32[] [] ("Analysis Results")) -> ()  [unwired: 2 in, 2 out]
      }
      frame "Cancel" {
        n99 = property on="Analysis Results" class="MCListbox (strict)"("ItemNames"=string[][] [] ("Item Names"), "Value"=i32[] [] ("Analysis Results")) -> ()  [unwired: 2 in, 2 out]
      }
      frame "UpdateSymbol" {
      }
      frame "UpdateOrderInTable" {
        n100 = property on="SelectionList" class="Arr (strict)"() -> ("Value"=w213:T4[])  [unwired: 2 in, 2 out]
        n101 = property on="AnalysisResultNum" class="DigNum (strict)"() -> ("Value"=w212:i32)  [unwired: 2 in, 2 out]
        n102 = property on="Analysis Results" class="MCListbox (strict)"() -> ("ItemNames"=w215:string[][])  [unwired: 2 in, 2 out]
        n103 = call "SelectionListToOrder.vi"("AnalysisResultNum"=w212, "SelectionList"=w213) -> ("Order"=w211:i32[])  [unwired: 9 in]
        n104 = for {
          tunnel: w211 -> [w229]
          tunnel: w215 -> [w227] mode=indexing
          tunnel: [w226] -> w214 mode=indexing
          tunnel: [w216] -> w210 mode=indexing
          i -> [w228]
          n105 = Search 1D Array(1D array=w229, element=w228) -> (index of element=w222:i32)  [unwired: 1 in]
          n106 = Increment(x=w222) -> (x+1=w220:i32)
          n107 = Less Than 0?(x=w222) -> (x < 0?=w219:bool)
          n108 = Number To Decimal String(number=w220) -> (decimal integer string=w221:string)  [unwired: 1 in]
          n109 = Select(t=" " ("new element/subarray"), s=w219, f=w221) -> (s? t:f=w223:string)
          n110 = Select(t=37 ("y"), s=w219, f=38 ("y")) -> (s? t:f=w216:i32)
          n111 = Replace Array Subset(array=w227, new element=w223, index=1) -> (w226:string[])
        }
        n112 = property on="Analysis Results" class="MCListbox (strict)"("ItemNames"=w214, "ItemSyms"=w210) -> ()  [unwired: 2 in, 2 out]
      }
      frame "UpdateAnalysisTable" {
        # "UpdateSelectionList"
        n113 = property on="SelectionList" class="Arr (strict)"() -> ("Value"=w237:T4[])  [unwired: 2 in, 2 out]
        n114 = property on="AnalysisResultNum" class="DigNum (strict)"() -> ("Value"=w233:i32)  [unwired: 2 in, 2 out]
        n115 = property on="Row" class="DigNum (strict)"() -> ("Value"=w234:i32)  [unwired: 2 in, 2 out]
        n116 = property on="Analysis Results" class="MCListbox (strict)"() -> ("ItemSyms"=w240:i32[])  [unwired: 2 in, 2 out]
        n117 = Less?(x=w234, y=w233) -> (x < y?=w235:bool)
        n118 = in-place {
          in-place-border: [w256] -> w238
          w260 = 37 ("y")
          # "UpdateSymbol"
          n119 = in-place-array #1(w240, w234) -> (w258:i32)
          n120 = Equal?(x=w258, y=w260) -> (x = y?=w256:bool)
          n121 = Select(t=38 ("y"), s=w256, f=w260) -> (s? t:f=w257:i32)
          n122 = in-place-array #1(w257) -> (w239:i32[])  [unwired: 1 out]
        }
        n123 = case shown="True" w235 {
          tunnel: w234 -> [w243 w246]
          tunnel: [w244 w247] -> w232
          tunnel: w233 -> [w242 _]
          frame False {
            n124 = Subtract(x=w243, y=w242) -> (x-y=w241:i32)
            n125 = Bundle("Type"=SelectionListEntryPointType."CaliperResult", w241) -> (w244:cluster{"Type":T5, i32})  [unwired: 1 in]
          }
          frame True {
            n126 = Bundle("Type"=SelectionListEntryPointType."AnalysisResult", "Value"=w246) -> (w247:cluster{"Type":T5, "Value":i32})  [unwired: 1 in]
          }
        }
        n127 = case shown="True" w238 {
          tunnel: w237 -> [w252 w255]
          tunnel: [w251 w254] -> w236
          tunnel: w232 -> [w249 w253]
          frame False {
            n128 = Search 1D Array(1D array=w252, element=w249) -> (index of element=w250:i32)  [unwired: 1 in]
            n129 = Delete From Array(array=w252, index=w250) -> (array with subset deleted=w251:T4[])  [unwired: 1 in, 1 out]
          }
          frame True {
            n130 = Build Array (concatenate)(w255, w253) -> (w254:T4[])
          }
        }
        n131 = property on="Analysis Results" class="MCListbox (strict)"("ItemSyms"=w239) -> ()  [unwired: 2 in, 2 out]
        n132 = property on="SelectionList" class="Arr (strict)"("Value"=w236) -> ()  [unwired: 2 in, 2 out]
      }
      frame "Run" {
        n133 = Not(x=w262) -> (.not. x?=w261:bool)
        n134 = call "[FGV] Analysis_Result_Points.vi"("CoordSystemRun"=w261, "Action"=AnalysisResultPointsAction."ReadAll") -> ("Analysis_Point_Result Out"=w280:T9[])  [unwired: 8 in, 1 out]
        n135 = call "[FGV] Analysis_Result_Points_Overlay.vi"("CoordSystemRun"=w261, "Action"=AnalysisResultPointsAction."ReadAll") -> ("Analysis_Point_Result Out"=w269:T9[])  [unwired: 8 in, 1 out]
        n136 = property on="CaliperEntryList" class="Arr (strict)"() -> ("Value"=w279:T2[])  [unwired: 2 in, 2 out]
        n137 = property on="CaliperEntryList Overlay" class="Arr (strict)"() -> ("Value"=w270:T2[])  [unwired: 2 in, 2 out]
        n138 = call "CaliperEntryFilter.vi"("CaliperEntryList"=w279) -> ("FilteredCaliperEntry"=w278:T11[])  [unwired: 10 in]
        n139 = call "CaliperEntryFilter.vi"("CaliperEntryList"=w270) -> ("FilteredCaliperEntry"=w268:T11[])  [unwired: 10 in]
        n140 = property on="SelectionList" class="Arr (strict)"() -> ("Value"=w267:T4[])  [unwired: 2 in, 2 out]
        n141 = call "Run Caliper.vi"("SelectionList"=w267, "FilteredCaliperEntry"=w278, "Analysis_Point_Result"=w280, "CaliperType"="CaliperType_w_Pic") -> ("error out"=w277:errorcluster, "Result"=w276:T1)  [unwired: 5 in, 1 out]
        n142 = call "Run Caliper.vi"("SelectionList"=w267, "FilteredCaliperEntry"=w268, "Analysis_Point_Result"=w269, "CaliperType"="CaliperType_w_Pic") -> ("error out"=w263:errorcluster, "Result"=w266:T1)  [unwired: 5 in, 1 out]
        n143 = case shown="No Error" w277 {
          selector: w277 -> [_ w291]
          tunnel: w276 -> [w285 w290]
          tunnel: "CaliperType_w_Pic" -> [w283 _]
          tunnel: [w285 w290] -> w275
          tunnel: [w284 w287] -> w274
          tunnel: w266 -> [w282 _]
          tunnel: [w282 _] -> w265
          tunnel: w263 -> [_ w286]
          frame No Error {
            n144 = call "CaliperResultToString.vi"("Result"=w285, "CaliperType_w_Pic"=w283) -> ("ResultString"=w284:string)  [unwired: 9 in]
            n145 = call "CaliperResultToString.vi"("Result"=w282, "CaliperType_w_Pic"=w283) -> ()  [unwired: 9 in, 1 out]
          }
          frame Error {
            n146 = Unbundle By Name(w291) -> ("source"=w288:string)
            n147 = call <vilib>:"Clear Errors.vi"("error in (no error)"=w286) -> ()  [unwired: 5 in, 2 out]
            n148 = Concatenate Strings("Error~!!!", w288) -> (w287:string)
          }
        }
        "Result" <- w275
        "Result Overlay" <- w265
        n149 = property on="Result" class="Str"("Value"=w274) -> ()  [unwired: 2 in, 2 out]
      }
      frame "AddCaliperEntry" {
        n150 = Not(x=w293) -> (.not. x?=w292:bool)
        n151 = call "[FGV] Analysis_Result_Points.vi"("CoordSystemRun"=w292, "Action"=AnalysisResultPointsAction."ReadAll") -> ("Analysis_Point_Result Out"=w309:T9[])  [unwired: 8 in, 1 out]
        n152 = call "[FGV] Analysis_Result_Points_Overlay.vi"("CoordSystemRun"=w292, "Action"=AnalysisResultPointsAction."ReadAll") -> ("Analysis_Point_Result Out"=w297:T9[])  [unwired: 8 in, 1 out]
        n153 = property on="CaliperEntryList" class="Arr (strict)"() -> ("Value"=w305:T2[])  [unwired: 2 in, 2 out]
        n154 = property on="CaliperEntryList Overlay" class="Arr (strict)"() -> ("Value"=w300:T2[])  [unwired: 2 in, 2 out]
        n155 = call "CaliperEntryFilter.vi"("CaliperEntryList"=w305) -> ("FilteredCaliperEntry"=w304:T11[])  [unwired: 10 in]
        n156 = call "CaliperEntryFilter.vi"("CaliperEntryList"=w300) -> ("FilteredCaliperEntry"=w299:T11[])  [unwired: 10 in]
        n157 = local read "CaliperType_w_Pic"() -> (w301:T6)
        n158 = property on="SelectionList" class="Arr (strict)"() -> ("Value"=w294:T4[])  [unwired: 2 in, 2 out]
        n159 = call "Run Caliper.vi"("SelectionList"=w294, "FilteredCaliperEntry"=w304, "Analysis_Point_Result"=w309, "CaliperType"=w301) -> ("error out"=w308:errorcluster, "SelectionListOut"=w306:T4[], "Result"=w307:T1)  [unwired: 5 in]
        n160 = call "Run Caliper.vi"("SelectionList"=w294, "FilteredCaliperEntry"=w299, "Analysis_Point_Result"=w297, "CaliperType"=w301) -> ("SelectionListOut"=w296:T4[], "Result"=w295:T1)  [unwired: 5 in, 1 out]
        n161 = case shown="No Error" w308 {
          selector: w308 -> [_ w327]
          tunnel: w307 -> [w314 _]
          tunnel: w306 -> [w320 _]
          tunnel: w301 -> [w313 _]
          tunnel: w296 -> [w311 _]
          tunnel: w295 -> [w312 _]
          frame No Error {
            n162 = Bundle By Name(cluster=T2 {"CaliperType"=0, "Points"=[], "Result"={"PointInclude?"=FALSE, "Num_Of_Pts"=0, "Position.X"=0.0, "Position.Y"=0.0, "Angle"=0.0, "Distance"=0.0, "Area"=0.0, "Radius_MAX"=0.0, "Radius2_min"=0.0, "Dev_Residual"=0.0, "P2.X"=0.0, "P2.Y"=0.0, "StepName"="", "Point ID"=0, "StepError?"=FALSE, "ResultDiff?"=FALSE}, "StepName"=""} ("CaliperEntry"), "Result"=w314, "Points"=w320, "CaliperType"=w313) -> (w319:T2)
            n163 = Bundle By Name(cluster=T2 {"CaliperType"=0, "Points"=[], "Result"={"PointInclude?"=FALSE, "Num_Of_Pts"=0, "Position.X"=0.0, "Position.Y"=0.0, "Angle"=0.0, "Distance"=0.0, "Area"=0.0, "Radius_MAX"=0.0, "Radius2_min"=0.0, "Dev_Residual"=0.0, "P2.X"=0.0, "P2.Y"=0.0, "StepName"="", "Point ID"=0, "StepError?"=FALSE, "ResultDiff?"=FALSE}, "StepName"=""} ("CaliperEntry"), "CaliperType"=w313, "Result"=w312, "Points"=w311) -> (w316:T2)
            n164 = property on="CaliperEntryList" class="Arr (strict)"() -> ("Value"=w323:T2[])  [unwired: 2 in, 2 out]
            n165 = property on="CaliperEntryList Overlay" class="Arr (strict)"() -> ("Value"=w317:T2[])  [unwired: 2 in, 2 out]
            n166 = Build Array (concatenate)(w323, w319) -> (w322:T2[])
            n167 = Build Array (concatenate)(w317, w316) -> (w315:T2[])
            n168 = property on="CaliperEntryList" class="Arr (strict)"("Value"=w322) -> ()  [unwired: 2 in, 2 out]
            n169 = property on="CaliperEntryList Overlay" class="Arr (strict)"("Value"=w315) -> ()  [unwired: 2 in, 2 out]
          }
          frame Error {
            n170 = Unbundle By Name(w327) -> ("source"=w325:string)
            n171 = Concatenate Strings("Cannot Add Caliper~!!!\nError Occurred for ", w325) -> (w324:string)
            n172 = One Button Dialog(message=w324) -> ()  [unwired: 1 in, 1 out]
          }
        }
      }
      frame "ReplaceCaliperEntry" {
        n173 = Not(x=w329) -> (.not. x?=w328:bool)
        n174 = call "[FGV] Analysis_Result_Points.vi"("CoordSystemRun"=w328, "Action"=AnalysisResultPointsAction."ReadAll") -> ("Analysis_Point_Result Out"=w346:T9[])  [unwired: 8 in, 1 out]
        n175 = property on="CaliperEntryList" class="Arr (strict)"() -> ("Value"=w348:T2[])  [unwired: 2 in, 2 out]
        n176 = property on="CaliperList" class="LstBox (strict)"() -> ("Value"=w335:i32)  [unwired: 2 in, 2 out]
        n177 = call "[FGV] Analysis_Result_Points_Overlay.vi"("CoordSystemRun"=w328, "Action"=AnalysisResultPointsAction."ReadAll") -> ("Analysis_Point_Result Out"=w332:T9[])  [unwired: 8 in, 1 out]
        n178 = property on="CaliperEntryList Overlay" class="Arr (strict)"() -> ("Value"=w336:T2[])  [unwired: 2 in, 2 out]
        n179 = Array Subset(array=w348, length=w335) -> (w349:T2[])  [unwired: 1 in]
        n180 = call "CaliperEntryFilter.vi"("CaliperEntryList"=w349) -> ("FilteredCaliperEntry"=w341:T11[])  [unwired: 10 in]
        n181 = Array Subset(array=w336, length=w335) -> (w334:T2[])  [unwired: 1 in]
        n182 = local read "CaliperType_w_Pic"() -> (w338:T6)
        n183 = call "CaliperEntryFilter.vi"("CaliperEntryList"=w334) -> ("FilteredCaliperEntry"=w333:T11[])  [unwired: 10 in]
        n184 = property on="SelectionList" class="Arr (strict)"() -> ("Value"=w345:T4[])  [unwired: 2 in, 2 out]
        n185 = call "Run Caliper.vi"("SelectionList"=w345, "FilteredCaliperEntry"=w341, "Analysis_Point_Result"=w346, "CaliperType"=w338) -> ("error out"=w344:errorcluster, "SelectionListOut"=w342:T4[], "Result"=w343:T1)  [unwired: 5 in]
        n186 = call "Run Caliper.vi"("FilteredCaliperEntry"=w333, "Analysis_Point_Result"=w332, "CaliperType"=w338) -> ("SelectionListOut"=w331:T4[], "Result"=w330:T1)  [unwired: 6 in, 1 out]
        n187 = case shown="No Error" w344 {
          selector: w344 -> [_ w367]
          tunnel: w343 -> [w352 _]
          tunnel: w342 -> [w351 _]
          tunnel: w338 -> [w350 _]
          tunnel: w335 -> [w357 _]
          tunnel: w331 -> [w354 _]
          tunnel: w330 -> [w353 _]
          frame No Error {
            n188 = Bundle By Name(cluster=T2 {"CaliperType"=0, "Points"=[], "Result"={"PointInclude?"=FALSE, "Num_Of_Pts"=0, "Position.X"=0.0, "Position.Y"=0.0, "Angle"=0.0, "Distance"=0.0, "Area"=0.0, "Radius_MAX"=0.0, "Radius2_min"=0.0, "Dev_Residual"=0.0, "P2.X"=0.0, "P2.Y"=0.0, "StepName"="", "Point ID"=0, "StepError?"=FALSE, "ResultDiff?"=FALSE}, "StepName"=""} ("CaliperEntry"), "Result"=w352, "Points"=w351, "CaliperType"=w350) -> (w360:T2)
            n189 = Bundle By Name(cluster=T2 {"CaliperType"=0, "Points"=[], "Result"={"PointInclude?"=FALSE, "Num_Of_Pts"=0, "Position.X"=0.0, "Position.Y"=0.0, "Angle"=0.0, "Distance"=0.0, "Area"=0.0, "Radius_MAX"=0.0, "Radius2_min"=0.0, "Dev_Residual"=0.0, "P2.X"=0.0, "P2.Y"=0.0, "StepName"="", "Point ID"=0, "StepError?"=FALSE, "ResultDiff?"=FALSE}, "StepName"=""} ("CaliperEntry"), "CaliperType"=w350, "Result"=w353, "Points"=w354) -> (w356:T2)
            n190 = property on="CaliperEntryList" class="Arr (strict)"() -> ("Value"=w363:T2[])  [unwired: 2 in, 2 out]
            n191 = property on="CaliperEntryList Overlay" class="Arr (strict)"() -> ("Value"=w358:T2[])  [unwired: 2 in, 2 out]
            n192 = Replace Array Subset(array=w363, new element=w360, index=w357) -> (w362:T2[])
            n193 = Replace Array Subset(array=w358, new element=w356, index=w357) -> (w355:T2[])
            n194 = property on="CaliperEntryList Overlay" class="Arr (strict)"("Value"=w355) -> ()  [unwired: 2 in, 2 out]
            n195 = property on="CaliperEntryList" class="Arr (strict)"("Value"=w362) -> ()  [unwired: 2 in, 2 out]
          }
          frame Error {
            n196 = Unbundle By Name(w367) -> ("source"=w365:string)
            n197 = Concatenate Strings("Cannot Replace Caliper~!!!\nError Occurred for ", w365) -> (w364:string)
            n198 = One Button Dialog(message=w364) -> ()  [unwired: 1 in, 1 out]
          }
        }
      }
      frame "SetCaliperStepName" {
        n199 = property on="CaliperEntryList" class="Arr (strict)"() -> ("Value"=w372:T2[])  [unwired: 2 in, 2 out]
        n200 = for {
          tunnel: w372 -> [w379] mode=indexing
          tunnel: [w377] -> w371 mode=indexing
          tunnel: w368 -> [w376]
          i -> [w383]
          n201 = Unbundle By Name(w379) -> ("CaliperType"=w384:T3)
          n202 = Number To Decimal String(number=w383) -> (decimal integer string=w382:string)  [unwired: 1 in]
          n203 = case shown="12" w384 {
            tunnel: ["Dist" "MidP" "PerProj" "LinInter" "AngForHor" "AngFroVer" "AngDefBy3Poi" "AngDefBy4Poi" "BisectLine" "MidLine" "LineFit" "CircleFit" "Area"] -> w380
            frame 0, Default {
            }
            frame 1 {
            }
            frame 2 {
            }
            frame 3 {
            }
            frame 4 {
            }
            frame 5 {
            }
            frame 6 {
            }
            frame 7 {
            }
            frame 8 {
            }
            frame 9 {
            }
            frame 11 {
            }
            frame 12 {
            }
            frame 10 {
            }
          }
          n204 = Select(t="Coord_Cal_#", s=w376, f="Caliper") -> (s? t:f=w374:string)
          n205 = Concatenate Strings(w374, w382, "_" ("string"), w380) -> (w378:string)
          n206 = Bundle By Name(cluster=w379, "StepName"=w378) -> (w377:T2)
        }
        n207 = property on="CaliperEntryList" class="Arr (strict)"("Value"=w371) -> ()  [unwired: 2 in, 2 out]
      }
      frame "UpdateCaliperResultToTable" {
        # "For Reference, Need to Modify"
        n208 = property on="Analysis Results" class="MCListbox (strict)"() -> ("ItemNames"=w404:string[][])  [unwired: 2 in, 2 out]
        n209 = property on="CaliperEntryList" class="Arr (strict)"() -> ("Value"=w405:T2[])  [unwired: 2 in, 2 out]
        n210 = property on="AnalysisResultNum" class="DigNum (strict)"() -> ("Value"=w400:i32)  [unwired: 2 in, 2 out]
        n211 = call "CaliperEntryFilter.vi"("CaliperEntryList"=w405) -> ("FilteredCaliperEntry"=w403:T11[])  [unwired: 10 in]
        n212 = call "GetItemNames.vi"("AnalysisResultNum"=w400, "FilteredCaliperEntry"=w403, "Item Names"=w404) -> ("NameTagToAdd"=w401:string[], "Action"=w402:enum16{"None", "Add", "Delete"})  [unwired: 7 in]
        n213 = case shown="\"Delete\"" w402 {
          tunnel: w401 -> [w408 w428 w440]
          tunnel: w400 -> [w410 _ _]
          frame "None", Default {
            # "Replace會用到"
            n214 = property on="CaliperList" class="LstBox (strict)"() -> ("Value"=w409:i32)  [unwired: 2 in, 2 out]
            n215 = for {
              tunnel: w408 -> [w427] mode=indexing
              tunnel: [w425] -> w415 mode=indexing
              n216 = Match Pattern(string=w427, regular expression="_") -> (before substring=w425:string)  [unwired: 1 in, 3 out]
            }
            n217 = Number To Decimal String(number=w409) -> (decimal integer string=w417:string)  [unwired: 1 in]
            n218 = Decrement(x=w409) -> (x-1=w406:i32)
            n219 = Concatenate Strings("Caliper", w417) -> (w414:string)
            n220 = Search 1D Array(1D array=w415, element=w414) -> (index of element=w412:i32)  [unwired: 1 in]
            n221 = Index Array(array=w408, index=w406) -> (element=w407:string)
            n222 = Greater Or Equal To 0?(x=w412) -> (x >= 0?=w413:bool)
            n223 = Add(x=w412, y=w410) -> (x+y=w411:i32)
            n224 = case shown="True" w413 {
              tunnel: w411 -> [_ w420]
              tunnel: w407 -> [_ w419]
              frame False {
              }
              frame True {
                n225 = property on="Analysis Results" class="MCListbox (strict)"() -> ("ItemNames"=w423:string[][], "Value"=w421:i32[], "ItemSyms"=w422:i32[])  [unwired: 2 in, 2 out]
                n226 = Build Array(w419) -> (w418:string[])
                n227 = Replace Array Subset(array=w423, new element=w418, index (row)=w420) -> (w424:string[][])  [unwired: 1 in]
                n228 = property on="Analysis Results" class="MCListbox (strict)"("ItemNames"=w424, "Value"=w421, "ItemSyms"=w422) -> ()  [unwired: 2 in, 2 out]
              }
            }
          }
          frame "Add" {
            n229 = for {
              tunnel: w428 -> [w429] mode=indexing
              n230 = property on="Analysis Results" class="MCListbox (strict)"() -> ("ItemNames"=w430:string[][], "Value"=w433:i32[], "ItemSyms"=w434:i32[])  [unwired: 2 in, 2 out]
              n231 = Build Array(w429) -> (w431:string[])
              n232 = Build Array (concatenate)(w430, w431) -> (w432:string[][])
              n233 = Build Array (concatenate)(w434, 37) -> (w436:i32[])
              n234 = property on="Analysis Results" class="MCListbox (strict)"("ItemNames"=w432, "Value"=w433, "ItemSyms"=w436) -> ()  [unwired: 2 in, 2 out]
            }
          }
          frame "Delete" {
            n235 = for {
              tunnel: w440 -> [w444] mode=indexing
              tunnel: [w442] -> w438 mode=indexing
              tunnel: [37] -> w437 mode=indexing
              n236 = Build Array(w444, "") -> (w442:string[])
            }
            n237 = property on="Analysis Results" class="MCListbox (strict)"("ItemNames"=w438, "Value"=i32[] [] ("Analysis Results"), "ItemSyms"=w437) -> ()  [unwired: 2 in, 2 out]
          }
        }
      }
      frame "UpdateCaliperList" {
        n238 = property on="CaliperEntryList" class="Arr (strict)"() -> ("Value"=w448:T2[])  [unwired: 2 in, 2 out]
        n239 = for {
          tunnel: w448 -> [w453] mode=indexing
          tunnel: [w449] -> w447 mode=indexing
          n240 = Unbundle By Name(w453) -> ("CaliperType"=w452:T3, "Result"=w451:T1, "StepName"=w450:string)  [unwired: 1 out]
          n241 = disable-structure shown="Disabled" {
            disable-tunnel: w452 -> [w456 _]
            disable-tunnel: w451 -> [w455 _]
            disable-tunnel: w450 -> [w454 w457]
            disable-tunnel: [_ w457] -> w449
            frame Disabled {
              n242 = case shown="0, Default" w456 {
                tunnel: w455 -> [_ _]
                tunnel: w454 -> [_ _]
                frame 0, Default {
                }
                frame 1 {
                }
              }
            }
            frame Enabled {
            }
          }
        }
        n243 = property on="CaliperList" class="LstBox (strict)"("Item Names"=w447) -> ()  [unwired: 2 in, 2 out]
      }
      frame "RemoveCaliperEntry" {
        n244 = property on="AnalysisResultNum" class="DigNum (strict)"() -> ("Value"=w460:i32)  [unwired: 2 in, 2 out]
        n245 = property on="CaliperEntryList" class="Arr (strict)"() -> ("Value"=w466:T2[])  [unwired: 2 in, 2 out]
        n246 = property on="Analysis Results" class="MCListbox (strict)"() -> ("ItemNames"=w462:string[][])  [unwired: 2 in, 2 out]
        n247 = property on="CaliperList" class="LstBox (strict)"() -> ("Value"=w464:i32, "Item Names"=w465:string[])  [unwired: 2 in, 2 out]
        n248 = Index Array(array=w465, index=w464) -> (element=w463:string)
        n249 = Array Subset(array=w462, index (row)=w460) -> (w461:string[][])  [unwired: 3 in]
        n250 = call "RemoveCaliperEntry.vi"("CaliperListName"=w463, "AnalysisResult"=w461, "CaliperList"=w464, "CaliperEntryList"=w466) -> ("CaliperEntryList Out"=w467:T2[])  [unwired: 7 in]
        n251 = property on="CaliperEntryList" class="Arr (strict)"("Value"=w467) -> ()  [unwired: 2 in, 2 out]
      }
      frame "ResetSelectionList" {
        n252 = property on="Analysis Results" class="MCListbox (strict)"() -> ("ItemSyms"=w471:i32[])  [unwired: 2 in, 2 out]
        n253 = for {
          tunnel: w471 -> [_] mode=indexing
          tunnel: [37 ("y")] -> w472 mode=indexing
        }
        n254 = property on="Analysis Results" class="MCListbox (strict)"("ItemSyms"=w472) -> ()  [unwired: 2 in, 2 out]
        n255 = property on="SelectionList" class="Arr (strict)"("Value"=T4[] [] ("SelectionList")) -> ()  [unwired: 2 in, 2 out]
        n256 = property on="CaliperList" class="LstBox (strict)"("Value"=-1 ("CaliperList")) -> ()  [unwired: 2 in, 2 out]
      }
      frame "RunAll" {
        n257 = Not(x=w476) -> (.not. x?=w475:bool)
        n258 = call "[FGV] Analysis_Result_Points.vi"("CoordSystemRun"=w475, "Action"=AnalysisResultPointsAction."ReadAll") -> ("Analysis_Point_Result Out"=w484:T9[])  [unwired: 8 in, 1 out]
        n259 = property on="CaliperEntryList" class="Arr (strict)"() -> ("Value"=w486:T2[])  [unwired: 2 in, 2 out]
        n260 = property on="CaliperEntryList Overlay" class="Arr (strict)"() -> ("Value"=w480:T2[])  [unwired: 2 in, 2 out]
        n261 = call "[FGV] Analysis_Result_Points_Overlay.vi"("CoordSystemRun"=w475, "Action"=AnalysisResultPointsAction."ReadAll") -> ("Analysis_Point_Result Out"=w478:T9[])  [unwired: 8 in, 1 out]
        n262 = disable-structure shown="Enabled" {
          disable-tunnel: w486 -> [w489 w490]
          disable-tunnel: [w488 w490] -> w485
          frame Disabled {
            n263 = call "CaliperEntrySetToNone.vi"("CaliperEntryList"=w489) -> ("CaliperEntryOut"=w488:T2[])  [unwired: 9 in, 1 out]
          }
          frame Enabled {
          }
        }
        n264 = call "Run All Caliper Steps.vi"("Analysis_Point_Result"=w484, "CaliperEntryList"=w485) -> ("CaliperEntryOut"=w483:T2[])  [unwired: 9 in]
        n265 = call "Run All Caliper Steps.vi"("Analysis_Point_Result"=w478, "CaliperEntryList"=w480) -> ("CaliperEntryOut"=w477:T2[])  [unwired: 9 in]
        n266 = property on="CaliperEntryList Overlay" class="Arr (strict)"("Value"=w477) -> ()  [unwired: 2 in, 2 out]
        n267 = property on="CaliperEntryList" class="Arr (strict)"("Value"=w483) -> ()  [unwired: 2 in, 2 out]
      }
      frame "Updata Overlay" {
        n268 = Not(x=w492) -> (.not. x?=w491:bool)
        n269 = disable-structure shown="Enabled" {
          disable-tunnel: [w506 w509] -> w500
          disable-tunnel: w491 -> [_ w508]
          frame Disabled {
            n270 = call "[FGV] Analysis_Result_Points.vi"("Action"=AnalysisResultPointsAction."ReadAll") -> ("Analysis_Point_Result Out"=w506:T9[])  [unwired: 9 in, 1 out]
          }
          frame Enabled {
            n271 = call "[FGV] Analysis_Result_Points_Overlay.vi"("CoordSystemRun"=w508, "Action"=AnalysisResultPointsAction."ReadAll") -> ("Analysis_Point_Result Out"=w509:T9[])  [unwired: 8 in, 1 out]
          }
        }
        n272 = disable-structure shown="Enabled" {
          disable-tunnel: [w504 w505] -> w499
          frame Disabled {
            n273 = property on="CaliperEntryList" class="Arr (strict)"() -> ("Value"=w504:T2[])  [unwired: 2 in, 2 out]
          }
          frame Enabled {
            n274 = property on="CaliperEntryList Overlay" class="Arr (strict)"() -> ("Value"=w505:T2[])  [unwired: 2 in, 2 out]
          }
        }
        n275 = property on="SelectionList" class="Arr (strict)"() -> ("Value"=w497:T4[])  [unwired: 2 in, 2 out]
        n276 = local read "CaliperType_w_Pic"() -> (w501:T6)
        n277 = disable-structure shown="Enabled" {
          disable-tunnel: [w502 w503] -> w493
          frame Disabled {
            n278 = local read "Result"() -> (w502:T1)
          }
          frame Enabled {
            n279 = local read "Result Overlay"() -> (w503:T1)
          }
        }
        n280 = call "CaliperEntryFilter.vi"("CaliperEntryList"=w499) -> ("FilteredCaliperEntry"=w498:T11[])  [unwired: 10 in]
        n281 = call "Update Overlay.vi"("CaliperType_w_Pic"=w501, "Vision_Image 2"=w496, "Analysis_Point_Result Out"=w500, "FilteredCaliperEntry"=w498, "SelectionList 2"=w497, "Result 2"=w493) -> ("Image Out"=w494:T7)  [unwired: 9 in]
        n282 = local write "Vision_Image"(w494) -> ()
      }
      frame "Clean Overlay" {
        n283 = call "IMAQ Copy"("Image Dst"=w512, "Image Src"=w513) -> ("Image Dst Out"=w511:T7)  [unwired: 4 in, 1 out]
        n284 = local write "Vision_Image"(w513) -> ()
      }
    }
  }
  "Cancel?" <- w16
  n285 = disable-structure shown="Disabled" {
    frame Disabled {
      n286 = call "IMAQ Fit Line"() -> ()  [unwired: 6 in, 6 out]
      n287 = call "IMAQ Fit Circle 2"() -> ()  [unwired: 6 in, 6 out]
    }
    frame Enabled {
    }
  }
  n288 = Flush Queue(queue=w19) -> (queue out=w18:refnum<queue>, error out=w17:errorcluster)  [unwired: 1 in, 1 out]
  n289 = Release Queue(queue=w18, error in (no error)=w17) -> ()  [unwired: 1 in, 3 out]
